vi "enable_ctrls_by_label.vi"(6 "States":T1(array[ring])=[enum."Disabled and Grayed Out", enum."Enabled", enum."Enabled"], 7 "Names":string[](array[string]), 8 "error in":errorcluster, 9 "Refnum in":refnum<vi>) -> (0 "error out":errorcluster, 1 "Refnum out":refnum<vi>)   [LabVIEW 2016]
uses:
  <userlib>/_OpenG.lib/array/array.llb/Filter 1D Array (String)__ogtk.vi
panel:
  out "setup ID":u16
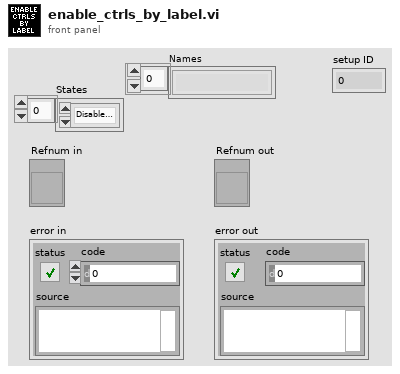
[diagram p1: front panel]
types:
  T1 = enum8{"Enabled", "Disabled", "Disabled and Grayed Out"}[]
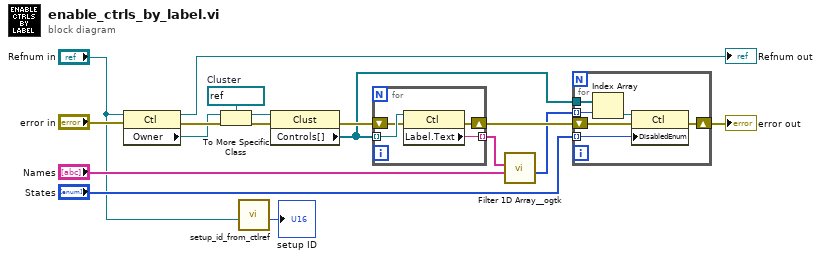
[diagram p0: block diagram]
diagram:
  w13 = refnum<vi> refnum  # Cluster
  n1 = property class="Ctl"(reference="Refnum in", error in="error in") -> (reference out=→"Refnum out":refnum<vi>, error out=w15:errorcluster, "Owner"=w14:refnum<vi>)
  n2 = To More Specific Class(target class=w13, reference=w14, error in=w15) -> (specific class reference=w12:refnum<vi>, error out=w11:errorcluster)
  n3 = call "setup_id_from_ctlref.vi"("Ctl Refnum"="Refnum in") -> ("setup ID"=→"setup ID":u16)  [unwired: 7 in, 1 out]
  n4 = property class="Clust"(reference=w12, error in=w11) -> (error out=w10:errorcluster, "Controls[]"=w7:refnum<vi>[])  [unwired: 1 out]
  n5 = for {
    tunnel: w7 -> [w21] mode=indexing
    tunnel: [w19] -> w9 mode=indexing
    shift-right: [w18] -> w5
    shift-left: w10 -> [w20]
    n6 = property class="Ctl"(reference=w21, error in=w20) -> (error out=w18:errorcluster, "Label.Text"=w19:string)  [unwired: 1 out]
  }
  n7 = call-poly <userlib>:"Filter 1D Array__ogtk.vi"("items to filter"="Names", "array"=w9) -> ("filtered item indices"=w3:i32[])  [unwired: 4 in, 1 out]
  n8 = for {
    tunnel: w3 -> [w26] mode=indexing
    tunnel: w7 -> [w27]
    tunnel: "States" -> [w24] mode=indexing
    shift-right: [w22] -> w4
    shift-left: w5 -> [w23]
    n9 = Index Array(array=w27, index=w26) -> (element=w25:refnum<vi>)
    n10 = property class="Ctl"(reference=w25, error in=w23, "DisabledEnum"=w24) -> (error out=w22:errorcluster)  [unwired: 1 out]
  }
  "error out" <- w4
